vi "Configure Trigger Bypass.vi"(8 "error in (no error)":errorcluster, 9 "Enable Trigger Layer Bypass (T:Enable)":bool=TRUE, 10 "Enable Arm Layer Bypass (T:Enable)":bool=TRUE, 11 "VISA resource name":refnum<visa-resource-name>) -> (0 "error out":errorcluster, 3 "VISA resource name out":refnum<visa-resource-name>)   [LabVIEW 2020, in "Keithley 24XX.lvlib"]
doc: "Configures settings for bypassing the triggering on the first iteration of a measurement."
uses:
  Keithley 24XX.lvlib
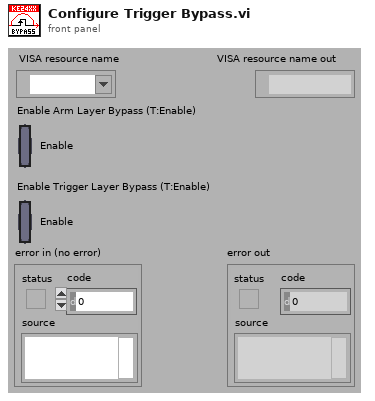
[diagram p1: front panel]
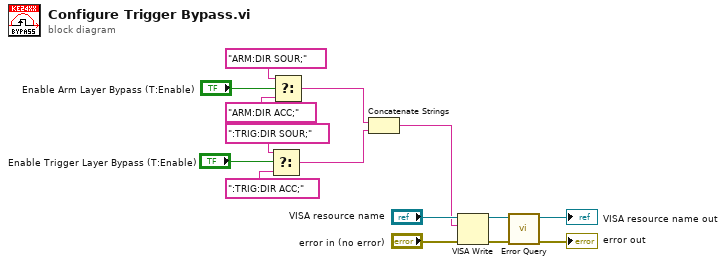
[diagram p0: block diagram]
diagram:
  n1 = Select(t=":TRIG:DIR SOUR;", s="Enable Trigger Layer Bypass (T:Enable)", f=":TRIG:DIR ACC;") -> (s? t:f=w2:string)
  n2 = Select(t="ARM:DIR SOUR;", s="Enable Arm Layer Bypass (T:Enable)", f="ARM:DIR ACC;") -> (s? t:f=w3:string)
  n3 = Concatenate Strings(w3, w2) -> (w1:string)
  n4 = VISA Write(VISA resource name="VISA resource name", write buffer=w1, error in (no error)="error in (no error)") -> (VISA resource name out=w11:refnum<visa-resource-name>, error out=w10:errorcluster)  [unwired: 1 out]
  n5 = call "Error Query.vi"("error in (no error)"=w10, "VISA resource name"=w11) -> ("error out"=→"error out":errorcluster, "VISA resource name out"=→"VISA resource name out":refnum<visa-resource-name>)  [unwired: 6 in, 2 out]
